vi "IMAQ FPGA CXP Counter1.vi"(10 "Reset":bool, 11 "Increment":bool) -> (3 "Count 1":u64)   [LabVIEW 2020]
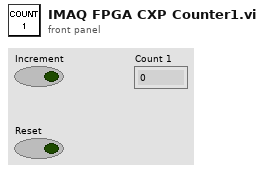
[diagram p1: front panel]
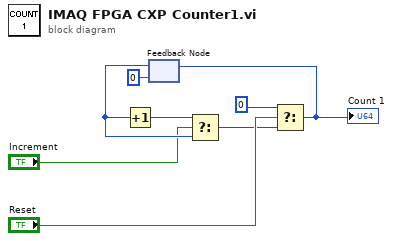
[diagram p0: block diagram]
diagram:
  n1 = feedback #1(u64 0) -> (w7:u64)
  n2 = Increment(x=w7) -> (x+1=w8:u64)
  n3 = Select(t=w8, s="Increment", f=w7) -> (s? t:f=w2:u64)
  n4 = Select(t=u64 0, s="Reset", f=w2) -> (s? t:f=w1:u64)
  "Count 1" <- w1
  n5 = feedback-in #1(w1) -> ()
